vi "LeastCommonMultiple.vi"(1 "Numeric (larger)":u32, 2 "Numeric":u32) -> (0 "LCM":u32)   [LabVIEW 2011]
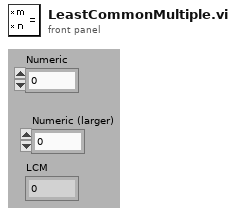
[diagram p1: front panel]
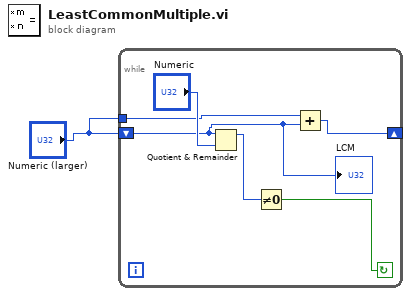
[diagram p0: block diagram]
diagram:
  n1 = while {
    shift-right: [w3] -> _
    shift-left: "Numeric (larger)" -> [w2]
    tunnel: "Numeric (larger)" -> [w4]
    stop <- w5 continue-if-true
    n2 = Quotient & Remainder(x=w2, y="Numeric") -> (x-y*floor(x/y)=w6:u32)  [unwired: 1 out]
    n3 = Not Equal To 0?(x=w6) -> (x != 0?=w5:bool)
    n4 = Add(x=w4, y=w2) -> (x+y=w3:u32)
    "LCM" <- w2
  }
